vi "AB_Engine_RESTful_Get_Class_Instantiation_Info.vi"(8 "error in (no error)":errorcluster, 11 "fully qualified LV class name":string[](array[string])) -> (0 "error out":errorcluster, 2 "qualified instantiation VI name":string, 3 "instantiation VI file name":string)   [LabVIEW 2020]
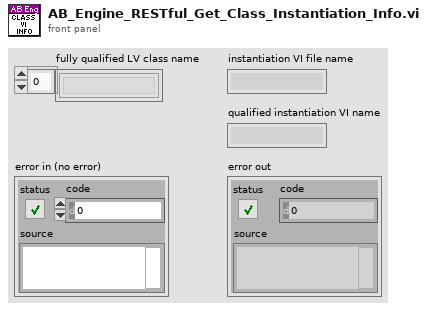
[diagram p1: front panel]
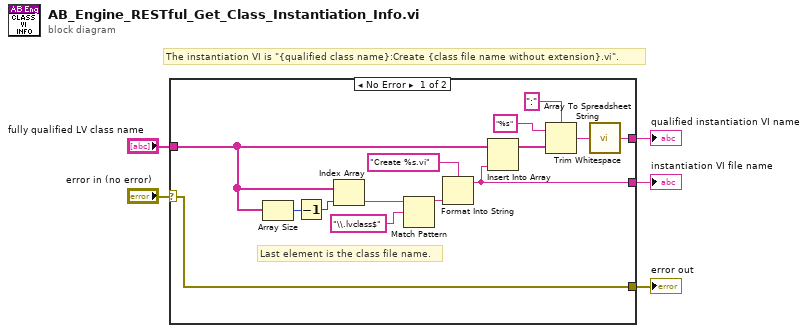
[diagram p0: block diagram]
diagram:
  # "The instantiation VI is \"{qualified class name}:Create {class file name without extension}.vi\"."
  n1 = case shown="No Error" "error in (no error)" {
    selector: "error in (no error)" -> [w18 w20]
    tunnel: [w19 _] -> w5
    tunnel: [w18 w20] -> w4
    tunnel: [w7 _] -> w3
    tunnel: "fully qualified LV class name" -> [w6 _]
    frame No Error {
      # "Last element is the class file name."
      n2 = Array Size(array=w6) -> (size(s)=w8:i32)
      n3 = Decrement(x=w8) -> (x-1=w9:i32)
      n4 = Index Array(array=w6, index=w9) -> (element=w10:string)
      n5 = Match Pattern(string=w10, regular expression="\\.lvclass$") -> (before substring=w12:string)  [unwired: 1 in, 3 out]
      n6 = Format Into String(format string="Create %s.vi", w12) -> (resulting string=w7:string)  [unwired: 2 in, 1 out]
      n7 = Insert Into Array(array=w6, new element=w7) -> (w14:string[])  [unwired: 1 in]
      n8 = Array To Spreadsheet String(delimiter (Tab)=":", array=w14, 3:"%s" ("format string")) -> (spreadsheet string=w17:string)
      n9 = call <vilib>:"Trim Whitespace.vi"("string"=w17) -> ("trimmed string"=w19:string)  [unwired: 1 in]
    }
    frame Error {
    }
  }
  "qualified instantiation VI name" <- w5
  "error out" <- w4
  "instantiation VI file name" <- w3
